vi "programa8.vi"() -> ()   [LabVIEW 2011]
panel:
  out "Contador":dbl
  out "Temp 36-60":dbl
  out "Temp 21-35":dbl
  out "Temp 1-20":dbl
  out "Temperatura":i32(slide) scale=0.0..60.0
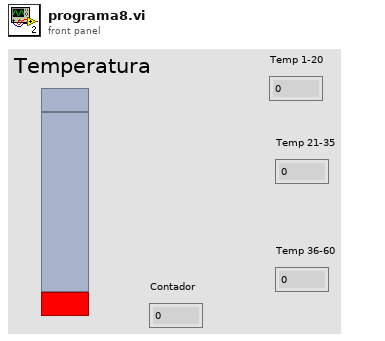
[diagram p1: front panel]
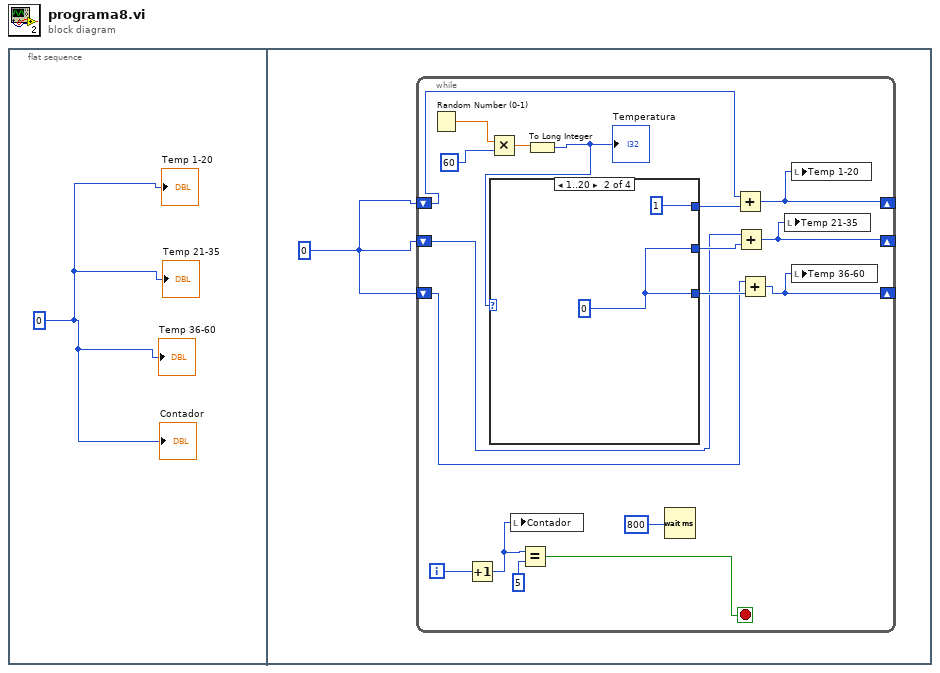
[diagram p0: block diagram]
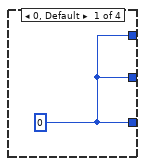
[diagram p2: hidden frame]
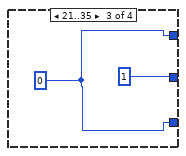
[diagram p3: hidden frame]
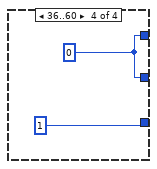
[diagram p4: hidden frame]
diagram:
  n1 = flat-sequence {
    frame #0 {
      w1 = 0
      "Temp 1-20" <- w1
      "Temp 21-35" <- w1
      "Temp 36-60" <- w1
      "Contador" <- w1
    }
    frame #1 {
      w2 = 0
      n2 = while {
        shift-right: [w5] -> _
        shift-left: w2 -> [w11]
        shift-right: [w4] -> _
        shift-left: w2 -> [w7]
        shift-right: [w3] -> _
        shift-left: w2 -> [w6]
        i -> [w20]
        stop <- w17 stop-if-true
        n3 = Random Number (0-1)() -> (number: 0 to 1=w15:dbl)
        n4 = Increment(x=w20) -> (x+1=w19:i32)
        n5 = Multiply(x=w15, y=60) -> (x*y=w13:dbl)
        n6 = local write "Contador"(w19) -> ()
        n7 = Equal?(x=w19, y=5) -> (x = y?=w17:bool)
        n8 = To Long Integer(number=w13) -> (32bit integer=w12:i32)
        "Temperatura" <- w12
        n9 = case shown="1..20" w12 {
          tunnel: [w21 1 w25 w26] -> w10
          tunnel: [w21 w23 1 w26] -> w9
          tunnel: [w21 w23 w25 1] -> w8
          frame 0, Default {
            w21 = 0
          }
          frame 1..20 {
            w23 = 0
          }
          frame 21..35 {
            w25 = 0
          }
          frame 36..60 {
            w26 = 0
          }
        }
        n10 = Wait (ms)(milliseconds to wait=800) -> ()  [unwired: 1 out]
        n11 = Add(x=w11, y=w10) -> (x+y=w5:i32)
        n12 = Add(x=w7, y=w9) -> (x+y=w4:i32)
        n13 = Add(x=w6, y=w8) -> (x+y=w3:i32)
        n14 = local write "Temp 21-35"(w4) -> ()
        n15 = local write "Temp 1-20"(w5) -> ()
        n16 = local write "Temp 36-60"(w3) -> ()
      }
    }
  }
